vi "MidbrainMain.vi"() -> ()   [LabVIEW 2012]
panel:
  in  "PortMotor":i32
  in  "StarboardMotor":i32
  in  "Notifiers":T1
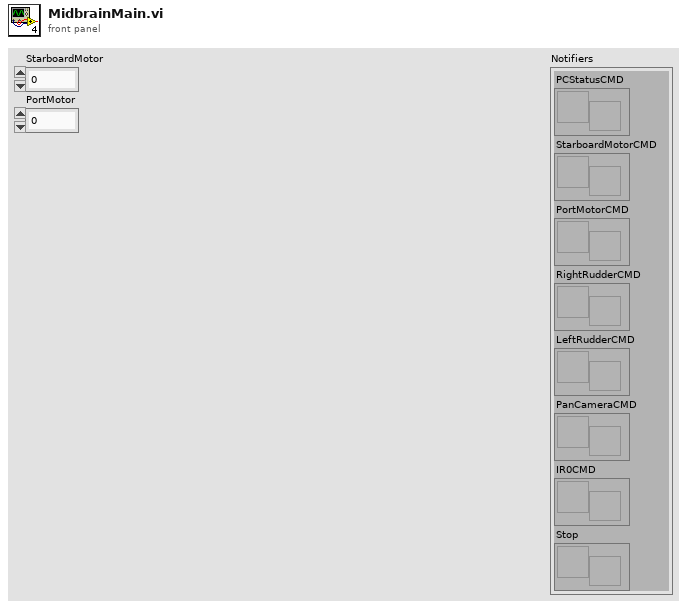
[diagram p1: front panel]
types:
  T1 = cluster{"PCStatusCMD":refnum<notifier>, "StarboardMotorCMD":refnum<notifier>, "PortMotorCMD":refnum<notifier>, "RightRudderCMD":refnum<notifier>, "LeftRudderCMD":refnum<notifier>, "PanCameraCMD":refnum<notifier>, "IR0CMD":refnum<notifier>, "Stop":refnum<notifier>}
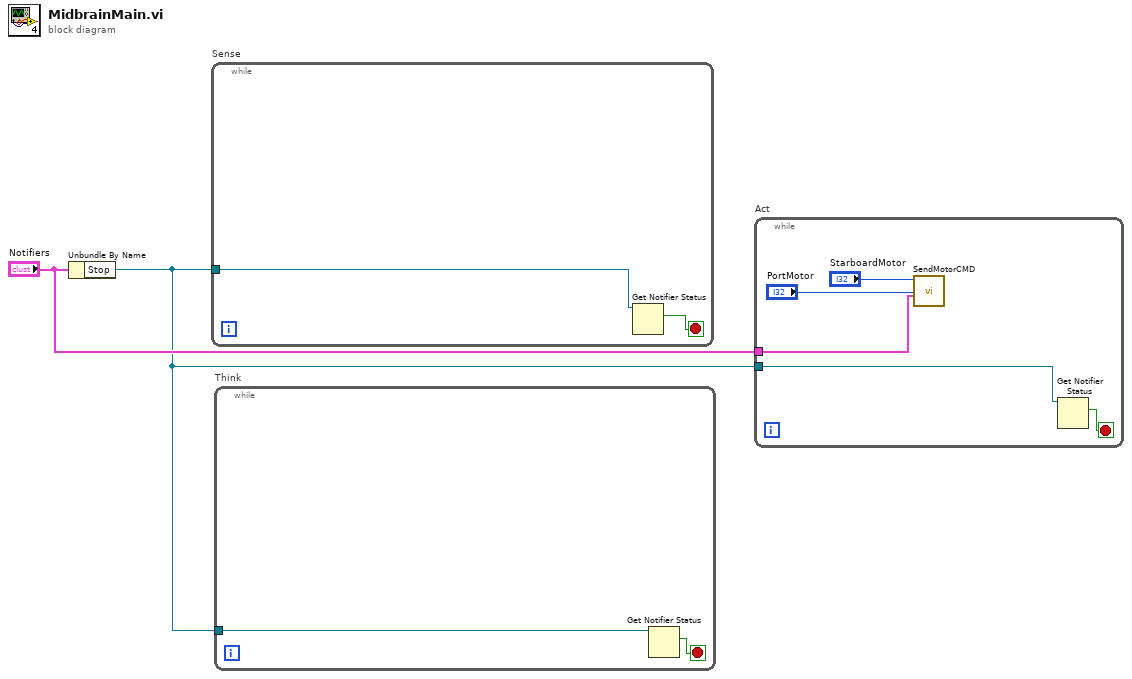
[diagram p0: block diagram]
diagram:
  n1 = Unbundle By Name("Notifiers") -> ("Stop"=w1:refnum<notifier>)
  n2 = while "Sense" {
    tunnel: w1 -> [w4]
    stop <- w3 stop-if-true
    n3 = Get Notifier Status(notifier=w4) -> (current notification=w3:bool)  [unwired: 1 in, 4 out]
  }
  n4 = while "Think" {
    tunnel: w1 -> [w6]
    stop <- w5 stop-if-true
    n5 = Get Notifier Status(notifier=w6) -> (current notification=w5:bool)  [unwired: 1 in, 4 out]
  }
  n6 = while "Act" {
    tunnel: w1 -> [w11]
    tunnel: "Notifiers" -> [w7]
    stop <- w10 stop-if-true
    n7 = call "SendMotorCMD.vi"("Notifiers"=w7, "PortMotor"="PortMotor", "StarboardMotor"="StarboardMotor") -> ()  [unwired: 2 in, 1 out]
    n8 = Get Notifier Status(notifier=w11) -> (current notification=w10:bool)  [unwired: 1 in, 4 out]
  }
